vi "Select USB device.vi"(0 "System no.":i32=1 min=1 max=4 step=1, 1 "DLL Interface":T1=4 items=["RS232", "GPIB", "Board", "TCP-IP", "USB", "RS232_DC", "USB_DC"], 2 "Controller name":string, 3 "Timeout":i32=5000, 5 "error in":errorcluster) -> (14 "Selected USB controller":string, 15 "DeviceID out":i32, 19 "error out":errorcluster)   [LabVIEW 2020]
doc: "Performs a broadcast, returns names of all controllers matching Controller name and lets the user select the appropriate controller from a ring control. VI will also stop if Cancel is TRUE.\n\nC-413: Controller name = \"C-413\", DLL Interface = USB\nC-866: Controller name = \"C-866\", DLL Interface = USB\nC-867: Controller name = \"C-867\", DLL Interface = USB\nC-877: Controller name = \"C-877\", DLL Interface = USB\nC-884: Controller name = \"C-884\", DLL Interface = USB\nC-885: Controller name = \"C-885\", DLL Interface = USB\nC-886: Controller name = \"C-886\", DLL Interface = USB\nC-891: Controller name = \"C-891\", DLL Interface = USB\nE-135: Controller name = \"E-135\", DLL Interface = USB\nE-517: Controller name = \"E-517\", DLL Interface = USB\nE-518: Controller name = E-518 , DLL Interface = USB\nE-709: Controller name = E-709 , DLL Interface = USB\nE-712: Controller name = E-712 , DLL Interface = USB\nE-725: Controller name = E-725 , DLL Interface = USB\nE-727: Controller name = E-727 , DLL Interface = USB\nE-754: Controller name = E-754 , DLL Interface = USB\nE-816: Controller name = \"E-816\", DLL Interface = USB\nE-861: Controller name = \"E-861\", DLL Interface = USB\nE-870: Controller name = \"E-870\", DLL Interface = USB\nE-871: Controller name = \"E-871\", DLL Interface = USB\nE-872: Controller name = \"E-872\", DLL Interface = USB\nE-873: Controller name = \"E-873\", DLL Interface = USB\nE-874: Controller name = \"E-874\", DLL Interface = USB\nMercury_GCS: Controller name = \"Mercury_GCS\", DLL Interface = USB"
uses:
  Available DLL interfaces.ctl
  Available interfaces.ctl
  Available DLLs.ctl
  Global1.vi
panel:
  in  "abort":bool
  in  "ok":bool
  in  "Please select USB controller":u16(ring)
  out "Please wait":string="Broadcast is running, please wait..."
  # "Scan parameters and controller name to search for:"
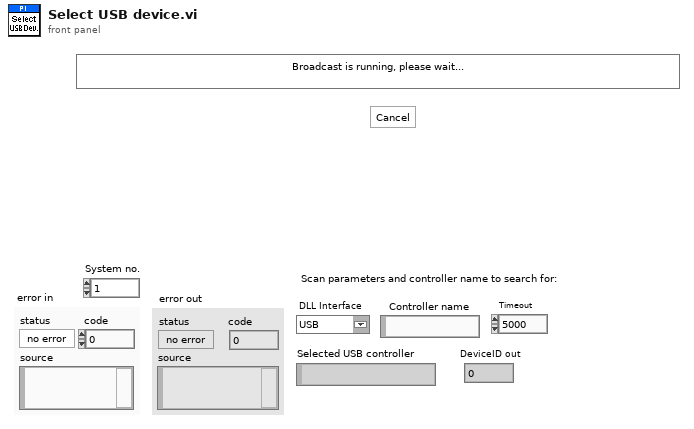
[diagram p1: front panel]
types:
  T1 = typedef "Available DLL interfaces.ctl" = u16
  T2 = enum16{"C844_IsDLLAvailable", "C844_ConnectRS232", "C844_ConnectNIgpib", "C844_IsConnected", "C844_CloseConnection", "C844_GcsCommandset", "C844_GetError", "C844_GcsGetAnswerSize", "C844_GcsGetAnswer", "C843_IsDLLAvailable", "C843_Connect", "C843_IsConnected", "C843_CloseConnection", "C843_GcsCommandset", "C843_GetError", "C843_GcsGetAnswerSize", "C843_GcsGetAnswer", "E710_IsDLLAvailable", "E710_ConnectRS232", "E710_ConnectNIgpib", "E710_IsConnected", "E710_CloseConnection", "E710_GcsCommandset", "E710_GetError", "E710_GcsGetAnswerSize", "E710_GcsGetAnswer", "C843_PM_IsDLLAvailable", "C843_PM_Connect", "C843_PM_IsConnected", "C843_PM_CloseConnection", "C843_PM_GcsCommandset", "C843_PM_GetError", "C843_PM_GcsGetAnswerSize", "C843_PM_GcsGetAnswer", "C843_PM_GetCurrentBoardID", "C843_GetCurrentBoardID", "C865_IsDLLAvailable", "C865_ConnectRS232", "C865_IsConnected", "C865_CloseConnection", "C865_GcsCommandset", "C865_GetError", "C865_GcsGetAnswerSize", "C865_GcsGetAnswer", "C865_GetCurrentInterfaceID", "E761_ConnectPciBoard", "DefineSystem", "CloseConnection", "IsConnected", "ConnectRS232", "ConnectNIgpib", "ConnectPciBoard", "ConnectTCPIP", "GetError", "GcsCommandset", "GCSGetAnswerSize", "GcsGetAnswer"}
  T3 = enum16{"C844_IsDLLAvailable", "C844_ConnectRS232", "C844_ConnectNIgpib", "C844_IsConnected", "C844_CloseConnection", "C844_GcsCommandset", "C844_GetError", "C844_GcsGetAnswerSize", "C844_GcsGetAnswer", "C843_IsDLLAvailable", "C843_Connect", "C843_IsConnected", "C843_CloseConnection", "C843_GcsCommandset", "C843_GetError", "C843_GcsGetAnswerSize", "C843_GcsGetAnswer", "E710_IsDLLAvailable", "E710_ConnectRS232", "E710_ConnectNIgpib", "E710_IsConnected", "E710_CloseConnection", "E710_GcsCommandset", "E710_GetError", "E710_GcsGetAnswerSize", "E710_GcsGetAnswer", "C843_PM_IsDLLAvailable", "C843_PM_Connect", "C843_PM_IsConnected", "C843_PM_CloseConnection", "C843_PM_GcsCommandset", "C843_PM_GetError", "C843_PM_GcsGetAnswerSize", "C843_PM_GcsGetAnswer", "C843_PM_GetCurrentBoardID", "C843_GetCurrentBoardID", "C865_IsDLLAvailable", "C865_ConnectRS232", "C865_IsConnected", "C865_CloseConnection", "C865_GcsCommandset", "C865_GetError", "C865_GcsGetAnswerSize", "C865_GcsGetAnswer", "C865_GetCurrentInterfaceID", "E761_ConnectPciBoard", "DefineSystem", "CloseConnection", "IsConnected", "ConnectRS232", "ConnectNIgpib", "ConnectPciBoard", "ConnectTCPIP", "GetError", "GcsCommandset", "GCSGetAnswerSize", "GcsGetAnswer", "CloseDaisyChain", "OpenRS232DaisyChain", "ConnectDaisyChainDevice", "ConnectUSB", "ListUSB"}
  T4 = typedef "Available DLLs.ctl" = u16
  T5 = typedef "Available interfaces.ctl" = u16
  T6 = cluster{"DLL for Device":T4, "DLL Interface":T1, "Parameter":string}[]
  T7 = cluster{"RS232 Portnumber":i32, "Timeout":i32, "RS232 Baud rate":u32, "Interface":T5, "GPIB Bus":i32, "GPIB Address":i32, "GPIB Mode":i32}[]
  T8 = cluster{"RS232 Portnumber":i32, "Timeout":i32, "RS232 Baud rate":u32, "Interface":T5, "GPIB Bus":i32, "GPIB Address":i32, "GPIB Mode":i32}
  T9 = cluster{"DLL for Device":T4, "DLL Interface":T1, "Parameter":string}
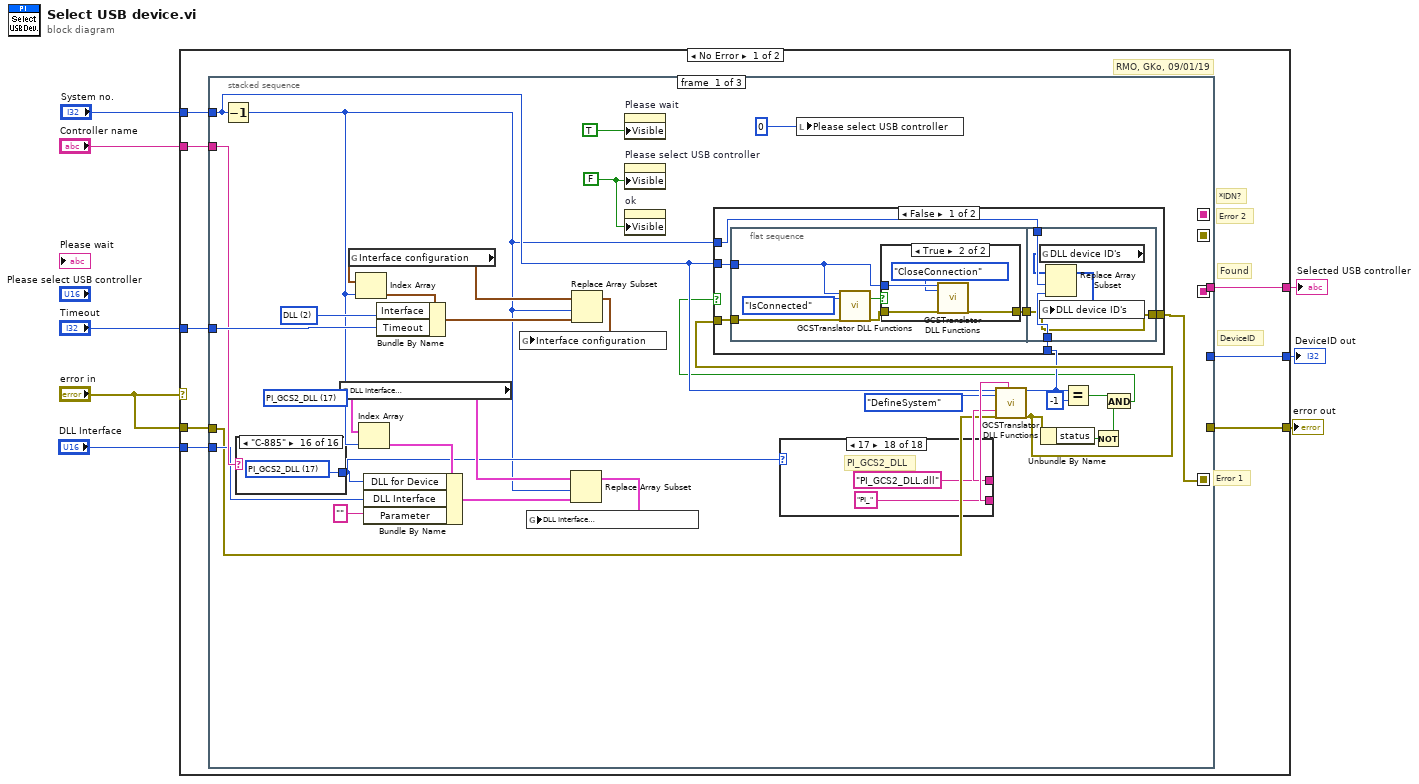
[diagram p0: block diagram]
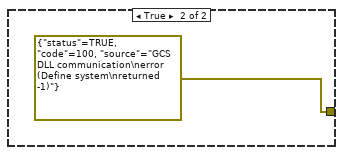
[diagram p3: hidden frame]
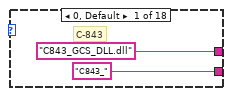
[diagram p4: hidden frame]
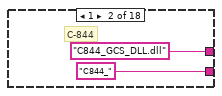
[diagram p5: hidden frame]
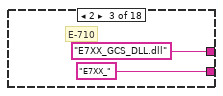
[diagram p6: hidden frame]
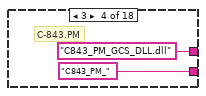
[diagram p7: hidden frame]
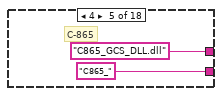
[diagram p8: hidden frame]
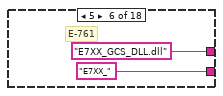
[diagram p9: hidden frame]
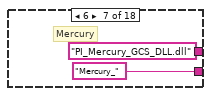
[diagram p10: hidden frame]
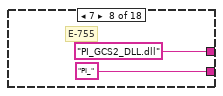
[diagram p11: hidden frame]
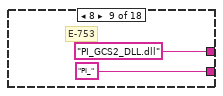
[diagram p12: hidden frame]
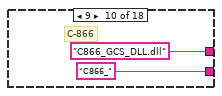
[diagram p13: hidden frame]
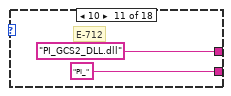
[diagram p14: hidden frame]
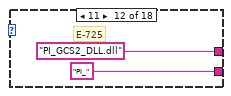
[diagram p15: hidden frame]
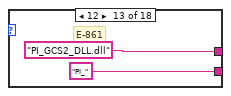
[diagram p16: hidden frame]
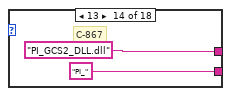
[diagram p17: hidden frame]
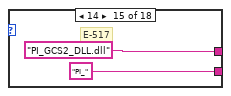
[diagram p18: hidden frame]
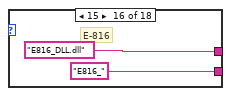
[diagram p19: hidden frame]
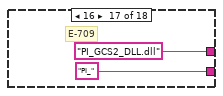
[diagram p20: hidden frame]
diagram:
  n1 = case shown="No Error" "error in" {
    tunnel: [w14 w253] -> w8
    tunnel: "error in" -> [w15 w253]
    tunnel: "Controller name" -> [w16 _]
    tunnel: [w13 "" ("Host address/name")] -> w5
    tunnel: [w12 0] -> w4
    tunnel: "System no." -> [w11 _]
    tunnel: "Timeout" -> [w10 _]
    tunnel: "DLL Interface" -> [w9 _]
    frame No Error {
      # "Error 1"
      # "DeviceID"
      # "Error 2"
      # "Found"
      # "*IDN?"
      # "RMO, GKo, 09/01/19"
      n2 = stacked-sequence {
        seq-local: [_ w126 _] -> [_ _ w201]
        seq-local: [_ w128 _] -> [_ _ w204]
        seq-local: [_ w125 _] -> [_ _ w199]
        seq-local: [w18 _ _] -> [_ w123 _]
        tunnel: w16 -> [w40 w127 _]
        tunnel: w15 -> [w22 _ _]
        tunnel: [_ _ w200] -> w14
        tunnel: [_ _ w203] -> w13
        tunnel: [_ _ w202] -> w12
        tunnel: w11 -> [w23 w124 _]
        tunnel: w10 -> [w44 _ _]
        tunnel: w9 -> [w39 _ _]
        frame #0 {
          (unwired) T4 17 items=["C-843", "C-844", "E-710", "C-843.PM", "C-865", "E-761", "Mercury", "E-755", "E-753", "C-866", "E-712", "E-725", "E-861", "C-867", "E-517", "E-816", "E-709", "PI_GCS2_DLL", "HydraPollux"] ("DLL for Device")
          w33 = FALSE ("Visible")
          w46 = T5 2 items=["RS232", "GPIB", "DLL", "TCP-IP"] ("Interface")
          n3 = Decrement(x=w23) -> (x-1=w20:i32)
          n4 = case shown="\"C-885\"" w40 {
            tunnel: [w107 w108 w109 w110 w111 w112 w113 w114 w115 w116 w117 w118 w119 w120 w121 w122] -> w27
            frame Default {
              w107 = T4 17 items=["C-843", "C-844", "E-710", "C-843.PM", "C-865", "E-761", "Mercury", "E-755", "E-753", "C-866", "E-712", "E-725", "E-861", "C-867", "E-517", "E-816", "E-709", "PI_GCS2_DLL", "HydraPollux"] ("DLL for Device")
            }
            frame "E-712" {
              w108 = T4 10 items=["C-843", "C-844", "E-710", "C-843.PM", "C-865", "E-761", "Mercury", "E-755", "E-753", "C-866", "E-712", "E-725", "E-861", "C-867", "E-517", "E-816", "E-709", "PI_GCS2_DLL", "HydraPollux"] ("DLL for Device")
            }
            frame "C-866" {
              w109 = T4 9 items=["C-843", "C-844", "E-710", "C-843.PM", "C-865", "E-761", "Mercury", "E-755", "E-753", "C-866", "E-712", "E-725", "E-861", "C-867", "E-517", "E-816", "E-709", "PI_GCS2_DLL", "HydraPollux"] ("DLL for Device")
            }
            frame "E-725" {
              w110 = T4 11 items=["C-843", "C-844", "E-710", "C-843.PM", "C-865", "E-761", "Mercury", "E-755", "E-753", "C-866", "E-712", "E-725", "E-861", "C-867", "E-517", "E-816", "E-709", "PI_GCS2_DLL", "HydraPollux"] ("DLL for Device")
            }
            frame "E-861" {
              w111 = T4 12 items=["C-843", "C-844", "E-710", "C-843.PM", "C-865", "E-761", "Mercury", "E-755", "E-753", "C-866", "E-712", "E-725", "E-861", "C-867", "E-517", "E-816", "E-709", "PI_GCS2_DLL", "HydraPollux"] ("DLL for Device")
            }
            frame "C-867" {
              w112 = T4 13 items=["C-843", "C-844", "E-710", "C-843.PM", "C-865", "E-761", "Mercury", "E-755", "E-753", "C-866", "E-712", "E-725", "E-861", "C-867", "E-517", "E-816", "E-709", "PI_GCS2_DLL", "HydraPollux"] ("DLL for Device")
            }
            frame "E-517" {
              w113 = T4 14 items=["C-843", "C-844", "E-710", "C-843.PM", "C-865", "E-761", "Mercury", "E-755", "E-753", "C-866", "E-712", "E-725", "E-861", "C-867", "E-517", "E-816", "E-709", "PI_GCS2_DLL", "HydraPollux"] ("DLL for Device")
            }
            frame "E-816" {
              w114 = T4 15 items=["C-843", "C-844", "E-710", "C-843.PM", "C-865", "E-761", "Mercury", "E-755", "E-753", "C-866", "E-712", "E-725", "E-861", "C-867", "E-517", "E-816", "E-709", "PI_GCS2_DLL", "HydraPollux"] ("DLL for Device")
            }
            frame "E-709" {
              w115 = T4 16 items=["C-843", "C-844", "E-710", "C-843.PM", "C-865", "E-761", "Mercury", "E-755", "E-753", "C-866", "E-712", "E-725", "E-861", "C-867", "E-517", "E-816", "E-709", "PI_GCS2_DLL", "HydraPollux"] ("DLL for Device")
            }
            frame "Mercury_GCS" {
              w116 = T4 17 items=["C-843", "C-844", "E-710", "C-843.PM", "C-865", "E-761", "Mercury", "E-755", "E-753", "C-866", "E-712", "E-725", "E-861", "C-867", "E-517", "E-816", "E-709", "PI_GCS2_DLL", "HydraPollux"] ("DLL for Device")
            }
            frame "C-884" {
              w117 = T4 17 items=["C-843", "C-844", "E-710", "C-843.PM", "C-865", "E-761", "Mercury", "E-755", "E-753", "C-866", "E-712", "E-725", "E-861", "C-867", "E-517", "E-816", "E-709", "PI_GCS2_DLL", "HydraPollux"] ("DLL for Device")
            }
            frame "C-877" {
              w118 = T4 17 items=["C-843", "C-844", "E-710", "C-843.PM", "C-865", "E-761", "Mercury", "E-755", "E-753", "C-866", "E-712", "E-725", "E-861", "C-867", "E-517", "E-816", "E-709", "PI_GCS2_DLL", "HydraPollux"] ("DLL for Device")
            }
            frame "E-871" {
              w119 = T4 17 items=["C-843", "C-844", "E-710", "C-843.PM", "C-865", "E-761", "Mercury", "E-755", "E-753", "C-866", "E-712", "E-725", "E-861", "C-867", "E-517", "E-816", "E-709", "PI_GCS2_DLL", "HydraPollux"] ("DLL for Device")
            }
            frame "C-413" {
              w120 = T4 17 items=["C-843", "C-844", "E-710", "C-843.PM", "C-865", "E-761", "Mercury", "E-755", "E-753", "C-866", "E-712", "E-725", "E-861", "C-867", "E-517", "E-816", "E-709", "PI_GCS2_DLL", "HydraPollux"] ("DLL for Device")
            }
            frame "E-870" {
              w121 = T4 17 items=["C-843", "C-844", "E-710", "C-843.PM", "C-865", "E-761", "Mercury", "E-755", "E-753", "C-866", "E-712", "E-725", "E-861", "C-867", "E-517", "E-816", "E-709", "PI_GCS2_DLL", "HydraPollux"] ("DLL for Device")
            }
            frame "C-885" {
              w122 = T4 17 items=["C-843", "C-844", "E-710", "C-843.PM", "C-865", "E-761", "Mercury", "E-755", "E-753", "C-866", "E-712", "E-725", "E-861", "C-867", "E-517", "E-816", "E-709", "PI_GCS2_DLL", "HydraPollux"] ("DLL for Device")
            }
          }
          n5 = global read "Global1.vi" "DLL Interface\nConfiguration"() -> (w35:T6)
          n6 = global read "Global1.vi" "Interface configuration"() -> (w36:T7)
          n7 = Index Array(array=w36, index=w20) -> (element=w47:T8)
          n8 = Index Array(array=w35, index=w20) -> (element=w45:T9)
          n9 = Bundle By Name(cluster=w45, "DLL for Device"=w27, "DLL Interface"=w39, "Parameter"="") -> (w37:T9)
          n10 = Bundle By Name(cluster=w47, "Interface"=w46, "Timeout"=w44) -> (w41:T8)
          n11 = Replace Array Subset(array=w35, new element=w37, index=w20) -> (w43:T6)
          n12 = global write "Global1.vi" "DLL Interface\nConfiguration"(w43) -> ()
          n13 = Replace Array Subset(array=w36, new element=w41, index=w20) -> (w42:T7)
          n14 = global write "Global1.vi" "Interface configuration"(w42) -> ()
          n15 = property on="Please wait" class="Str"("Visible"=TRUE) -> ()  [unwired: 2 in, 2 out]
          n16 = property on="Please select USB controller" class="Ring (strict)"("Visible"=w33) -> ()  [unwired: 2 in, 2 out]
          n17 = property on="ok" class="Bool"("Visible"=w33) -> ()  [unwired: 2 in, 2 out]
          n18 = case shown="17" w27 {
            tunnel: ["C843_GCS_DLL.dll" "C844_GCS_DLL.dll" "E7XX_GCS_DLL.dll" "C843_PM_GCS_DLL.dll" "C865_GCS_DLL.dll" "E7XX_GCS_DLL.dll" "PI_Mercury_GCS_DLL.dll" "PI_GCS2_DLL.dll" "PI_GCS2_DLL.dll" "C866_GCS_DLL.dll" "PI_GCS2_DLL.dll" "PI_GCS2_DLL.dll" "PI_GCS2_DLL.dll" "PI_GCS2_DLL.dll" "PI_GCS2_DLL.dll" "E816_DLL.dll" "PI_GCS2_DLL.dll" "PI_GCS2_DLL.dll"] -> w30
            tunnel: ["C843_" "C844_" "E7XX_" "C843_PM_" "C865_" "E7XX_" "Mercury_" "PI_" "PI_" "C866_" "PI_" "PI_" "PI_" "PI_" "PI_" "E816_" "PI_" "PI_"] -> w31
            frame 0, Default {
              # "C-843"
            }
            frame 1 {
              # "C-844"
            }
            frame 2 {
              # "E-710"
            }
            frame 3 {
              # "C-843.PM"
            }
            frame 4 {
              # "C-865"
            }
            frame 5 {
              # "E-761"
            }
            frame 6 {
              # "Mercury"
            }
            frame 7 {
              # "E-755"
            }
            frame 8 {
              # "E-753"
            }
            frame 9 {
              # "C-866"
            }
            frame 10 {
              # "E-712"
            }
            frame 11 {
              # "E-725"
            }
            frame 12 {
              # "E-861"
            }
            frame 13 {
              # "C-867"
            }
            frame 14 {
              # "E-517"
            }
            frame 15 {
              # "E-816"
            }
            frame 16 {
              # "E-709"
            }
            frame 17 {
              # "PI_GCS2_DLL"
            }
          }
          n19 = local write "Please select USB controller"(0) -> ()
          n20 = call "GCSTranslator DLL Functions.vi"("System no."=w23, "Function"=T2."DefineSystem", "String input"=w30, "error in"=w22, "String input 2"=w31) -> ("DLL I32 Return value"=w19:i32, "error out"=w21:errorcluster)  [unwired: 2 in, 11 out]
          n21 = Unbundle By Name(w21) -> ("status"=w25:bool)
          n22 = Equal?(x=w19, y=-1) -> (x = y?=w26:bool)
          n23 = Not(x=w25) -> (.not. x?=w24:bool)
          n24 = And(x=w26, y=w24) -> (x .and. y?=w17:bool)
          n25 = case shown="False" w17 {
            tunnel: w23 -> [w48 _]
            tunnel: w21 -> [w51 _]
            tunnel: w20 -> [w53 _]
            tunnel: w19 -> [w52 _]
            tunnel: [w49 errorcluster {"status"=TRUE, "code"=100, "source"="GCS DLL communication\nerror (Define system\nreturned -1)"} ("error out")] -> w18
            frame False {
              n26 = flat-sequence {
                tunnel: w51 -> [w56]
                tunnel: [w55] -> w50
                tunnel: w48 -> [w54]
                tunnel: w53 -> [w69]
                tunnel: w52 -> [w66]
                tunnel: w50 -> [w65]
                tunnel: [w65] -> w49
                frame #0 {
                  n27 = call "GCSTranslator DLL Functions.vi"("System no."=w54, "Function"=T2."IsConnected", "error in"=w56) -> ("Boolean output"=w59:bool, "error out"=w58:errorcluster)  [unwired: 4 in, 11 out]
                  n28 = case shown="True" w59 {
                    tunnel: w54 -> [_ w64]
                    tunnel: w58 -> [w60 w63]
                    tunnel: [w60 w62] -> w55
                    frame False {
                    }
                    frame True {
                      n29 = call "GCSTranslator DLL Functions.vi"("System no."=w64, "Function"=T2."CloseConnection", "error in"=w63) -> ("error out"=w62:errorcluster)  [unwired: 4 in, 12 out]
                    }
                  }
                }
                frame #1 {
                  n30 = global read "Global1.vi" "DLL device ID's"() -> (w67:i32[])
                  n31 = Replace Array Subset(array=w67, new element=w66, index=w69) -> (w68:i32[])
                  n32 = global write "Global1.vi" "DLL device ID's"(w68) -> ()
                }
              }
            }
            frame True {
            }
          }
        }
        frame #1 {
          n33 = case shown="No Error" w123 {
            tunnel: [w142 string[] []] -> w128
            tunnel: w127 -> [w130 _]
            tunnel: [w141 w198] -> w126
            tunnel: [w140 string[] []] -> w125
            tunnel: w124 -> [w134 _]
            tunnel: w123 -> [w132 w198]
            frame No Error {
              n34 = case shown="Default" w130 {
                tunnel: [w144 string[] ["C-663", "C-863"]] -> w129
                tunnel: w130 -> [w143 _]
                frame Default {
                  n35 = Build Array(w143) -> (w144:string[])
                }
                frame "Mercury_GCS" {
                }
              }
              n36 = call "GCSTranslator DLL Functions.vi"("System no."=w134, "Function"=T3."ListUSB", "error in"=w132) -> ("DLL I32 Return value"=w136:i32, "String output"=w133:string, "error out"=w139:errorcluster)  [unwired: 4 in, 10 out]
              n37 = call "Get lines from string.vi"("Input string"=w133) -> ("Strings"=w138:string[])  [unwired: 2 in, 16 out]
              n38 = Not Equal?(x=w136, y=-1) -> (x != y?=w137:bool)
              n39 = case shown="True" w137 {
                tunnel: [string[] [] w162] -> w142
                tunnel: [w146 w158] -> w141
                tunnel: [string[] [] w157] -> w140
                tunnel: w139 -> [w151 w156]
                tunnel: w138 -> [_ w155]
                tunnel: w134 -> [w150 _]
                tunnel: w129 -> [_ w154]
                frame False {
                  # "Error!"
                  n40 = call "GCSTranslator DLL Functions.vi"("System no."=w150, "Function"=T2."GetError", "error in"=w151) -> ("error out"=w147:errorcluster)  [unwired: 4 in, 12 out]
                  n41 = call "GCSTranslateError.vi"("error in"=w147) -> ("error out"=w146:errorcluster)  [unwired: 18 out]
                }
                frame True {
                  n42 = for {
                    tunnel: w155 -> [w167]
                    tunnel: w154 -> [w166] mode=indexing
                    shift-right: [w168] -> w157
                    shift-left: string[] [] -> [w165]
                    n43 = for {
                      tunnel: w167 -> [w172] mode=indexing
                      shift-right: [w171] -> w168
                      shift-left: w165 -> [w170]
                      tunnel: w166 -> [w169]
                      n44 = Match Pattern(string=w172, regular expression=w169) -> (offset past match=w175:i32)  [unwired: 4 out]
                      n45 = Not Equal?(x=w175, y=-1) -> (x != y?=w173:bool)
                      n46 = case shown="True" w173 {
                        tunnel: w172 -> [_ w177]
                        tunnel: [w176 w179] -> w171
                        tunnel: w170 -> [w176 w178]
                        frame False {
                        }
                        frame True {
                          n47 = Build Array (concatenate)(w178, w177) -> (w179:string[])
                        }
                      }
                    }
                  }
                  n48 = Array Size(array=w157) -> (size(s)=w161:i32)
                  n49 = Array Size(array=w157) -> (size(s)=w160:i32)
                  n50 = Equal To 0?(x=w160) -> (x = 0?=w159:bool)
                  n51 = Initialize Array("", w161) -> (w164:string[])
                  n52 = case shown="True" w159 {
                    tunnel: [w180 w182] -> w158
                    tunnel: w156 -> [w180 w181]
                    frame False {
                    }
                    frame True {
                      n53 = Bundle By Name(cluster=w181, "status"=TRUE, "code"=100 ("Bundle Element"), "source"="Controller not found" ("Bundle Element")) -> (w182:errorcluster)
                    }
                  }
                  n54 = for {
                    N: w161 -> [_]
                    shift-right: [w193] -> w162
                    shift-left: w164 -> [w195]
                    tunnel: w157 -> [w186] mode=indexing
                    i -> [w190]
                    n55 = Increment(x=w190) -> (x+1=w189:i32)
                    n56 = Number To Decimal String(number=w189, width (-)=i16 0) -> (decimal integer string=w188:string)
                    n57 = Concatenate Strings("DeviceID ", w188, ": " ("string"), w186) -> (w194:string)
                    n58 = Replace Array Subset(array=w195, new element=w194, index=w190) -> (w193:string[])
                  }
                }
              }
            }
            frame Error {
            }
          }
        }
        frame #2 {
          n59 = case shown="No Error" w201 {
            tunnel: w204 -> [w215 _]
            tunnel: w199 -> [w214 _]
            tunnel: [w213 "" ("Host address/name")] -> w203
            tunnel: [w211 0] -> w202
            tunnel: w201 -> [w209 w247]
            tunnel: [w205 w247] -> w200
            frame No Error {
              n60 = flat-sequence {
                tunnel: w215 -> [w217]
                tunnel: w209 -> [w216]
                tunnel: [w216] -> w208
                tunnel: w208 -> [w219]
                tunnel: [w219] -> w207
                tunnel: w214 -> [w225]
                tunnel: [w224] -> w212
                tunnel: [w223] -> w210
                tunnel: w207 -> [w222]
                tunnel: [w221] -> w206
                tunnel: [w246] -> w213
                tunnel: w212 -> [w246]
                tunnel: [w244] -> w211
                tunnel: w210 -> [w244]
                tunnel: [w243] -> w205
                tunnel: w206 -> [w243]
                frame #0 {
                  n61 = property on="Please wait" class="Str"("Visible"=FALSE) -> ()  [unwired: 2 in, 2 out]
                  n62 = property on="Please select USB controller" class="Ring (strict)"("Strings []"=w217) -> ()  [unwired: 2 in, 2 out]
                }
                frame #1 {
                  w220 = TRUE ("Visible")
                  n63 = property on="Please select USB controller" class="Ring (strict)"("Visible"=w220) -> ()  [unwired: 2 in, 2 out]
                  n64 = property on="ok" class="Bool"("Visible"=w220) -> ()  [unwired: 2 in, 2 out]
                }
                frame #2 {
                  n65 = while {
                    tunnel: w225 -> [w232]
                    tunnel: [w231] -> w224
                    tunnel: [w230] -> w223
                    tunnel: w222 -> [w229]
                    tunnel: [w228] -> w221
                    stop <- w234 stop-if-true
                    n66 = case shown="True" "abort" {
                      tunnel: w229 -> [w235 _]
                      tunnel: [w235 errorcluster {"status"=TRUE, "code"=100, "source"="Select USB device was canceled"} ("error out")] -> w228
                      frame False {
                      }
                      frame True {
                      }
                    }
                    n67 = case shown="True" "ok" {
                      tunnel: w232 -> [_ w242]
                      tunnel: ["" ("Host address/name") w241] -> w231
                      tunnel: [0 w239] -> w230
                      frame False {
                      }
                      frame True {
                        n68 = local read "Please select USB controller"() -> (w240:u16)
                        n69 = Increment(x=w240) -> (x+1=w239:u16)
                        n70 = Index Array(array=w242, index=w240) -> (element=w241:string)
                      }
                    }
                    n71 = Or(x="ok", y="abort") -> (x .or. y?=w234:bool)
                    n72 = Wait Until Next ms Multiple(millisecond multiple=u32 10) -> ()  [unwired: 1 out]
                  }
                }
                frame #3 {
                  n73 = local write "abort"(FALSE ("abort")) -> ()
                }
              }
            }
            frame Error {
              n74 = One Button Dialog(message="Error! \nController not found.\nPlease check settings and retry.") -> ()  [unwired: 2 out]
            }
          }
        }
      }
    }
    frame Error {
    }
  }
  "error out" <- w8
  "Selected USB controller" <- w5
  "DeviceID out" <- w4
